vi "Event Handler.vi"() -> ()   [LabVIEW 2024]
panel:
  out "current time":timestamp
  in  "Time Check":bool
  out "Iteration":i32
  in  "Stop":bool
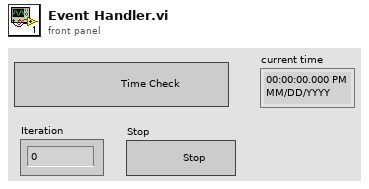
[diagram p1: front panel]
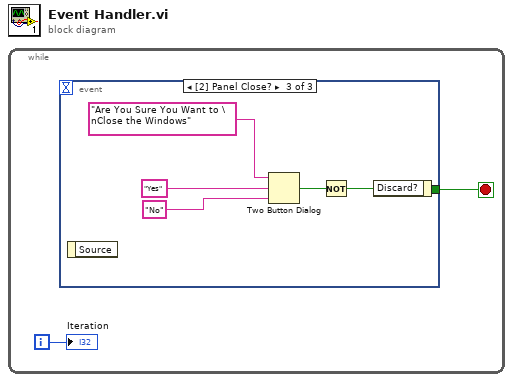
[diagram p0: block diagram]
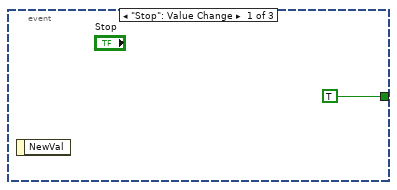
[diagram p2: hidden frame]
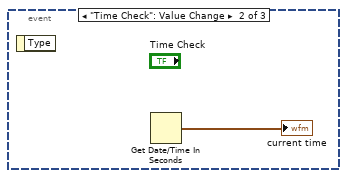
[diagram p3: hidden frame]
diagram:
  n1 = while {
    i -> [w2]
    stop <- w1 stop-if-true
    n2 = event shown="[2] Panel Close?" {
      selector: _ -> [_ _ _]
      dyn-events: _ -> [_ _ _]
      timeout: _ -> [_ _ _]
      tunnel: [TRUE _ _] -> w1
      event "Stop": Value Change {
        n3 = event-data() -> ()  [unwired: 1 in, 1 out]
      }
      event "Time Check": Value Change {
        n4 = event-data() -> ()  [unwired: 1 in, 1 out]
        n5 = Get Date/Time In Seconds() -> (seconds since 1Jan1904=→"current time":timestamp)
      }
      event Panel Close? {
        n6 = event-data() -> ()  [unwired: 1 in, 1 out]
        n7 = Two Button Dialog(message="Are You Sure You Want to \nClose the Windows", 1:"No", 2:"Yes") -> (T button?=w7:bool)
        n8 = Not(x=w7) -> (.not. x?=w6:bool)
        n9 = event-data("Discard?"=w6) -> ()  [unwired: 1 in, 1 out]
      }
    }
    "Iteration" <- w2
  }
